vi "Initialize.vi"(6 "Route(F)/Relay(T)":bool, 7 "Simulate?":bool, 8 "error in (no error)":errorcluster, 9 "Topology":string, 10 "Alias":string, 11 "Device/Resource Name":string) -> (0 "error out":errorcluster, 3 "PXI Card Config":refnum<class "PXI Card Config.lvclass">)   [LabVIEW 2018, in "PXI Card Config.lvclass"]
uses:
  Switch Configuration.llb/PXI Card Config.lvclass
  C:/Users/jennifer.platt/Documents/Switch-Custom-Device - Copy/Source/Switch Card Config/Switch Card Config.lvclass
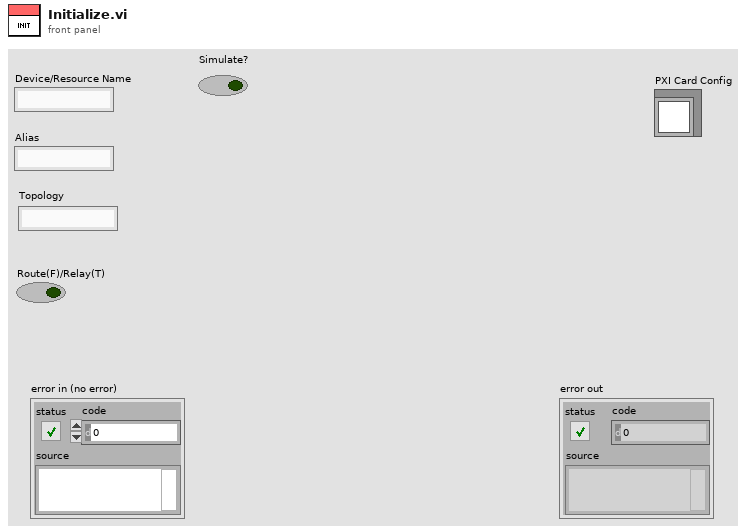
[diagram p1: front panel]
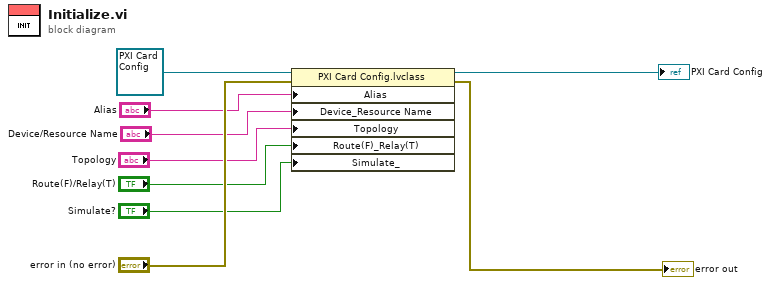
[diagram p0: block diagram]
diagram:
  n1 = property class="PXI Card Config.lvclass"(reference=refnum<class "PXI Card Config.lvclass"> refnum ("PXI Card Config"), error in="error in (no error)", "Alias"="Alias", "Device_Resource Name"="Device/Resource Name", "Topology"="Topology", "Route(F)_Relay(T)"="Route(F)/Relay(T)", "Simulate_"="Simulate?") -> (reference out=→"PXI Card Config":refnum<class "PXI Card Config.lvclass">, error out=→"error out":errorcluster)
